vi "Validate Address.vi"(11 "IP Address":string="localhost:50051") -> (3 "Valid":bool)   [LabVIEW 2020, in "gRPC Data Server System Explorer.lvlib"]
uses:
  gRPC Data Server System Explorer.lvlib
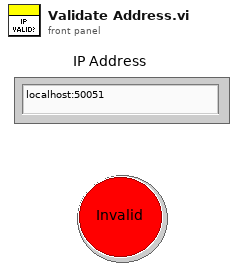
[diagram p1: front panel]
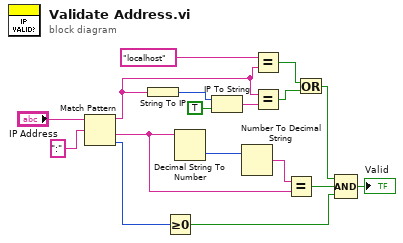
[diagram p0: block diagram]
diagram:
  n1 = Match Pattern(string="IP Address", regular expression=":") -> (before substring=w11:string, after substring=w2:string, offset past match=w12:i32)  [unwired: 1 in, 1 out]
  n2 = String To IP(1:w11) -> (0:w17:u32)
  n3 = Greater Or Equal To 0?(x=w12) -> (x >= 0?=w6:bool)
  n4 = Decimal String To Number(string=w2) -> (number=w4:i32)  [unwired: 2 in, 1 out]
  n5 = IP To String(1:TRUE ("dot notation? (F)"), 2:w17) -> (0:w15:string)
  n6 = Number To Decimal String(number=w4) -> (decimal integer string=w3:string)  [unwired: 1 in]
  n7 = Equal?(x="localhost", y=w11) -> (x = y?=w9:bool)
  n8 = Equal?(x=w11, y=w15) -> (x = y?=w8:bool)
  n9 = Equal?(x=w3, y=w2) -> (x = y?=w1:bool)
  n10 = Or(x=w9, y=w8) -> (x .or. y?=w7:bool)
  n11 = Compound Arithmetic op=AND(w7, w1, w6) -> (→"Valid":bool)
